vi "Check Python Version.vi"(11 "error in (no error)":errorcluster) -> (4 "standard output":string, 6 "Valid Version?":bool, 15 "error out":errorcluster)   [LabVIEW 2021, in "Measurement Builder.lvlib"]
uses:
  Measurement Builder.lvlib
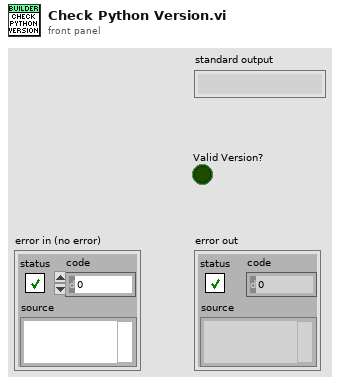
[diagram p1: front panel]
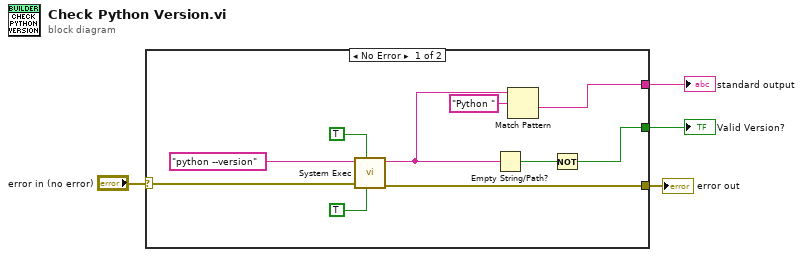
[diagram p0: block diagram]
diagram:
  n1 = case shown="No Error" "error in (no error)" {
    selector: "error in (no error)" -> [w11 w15]
    tunnel: [w10 w15] -> w4
    tunnel: [w5 _] -> w2
    tunnel: [w7 _] -> w1
    frame No Error {
      n2 = call <vilib>:"System Exec.vi"("run minimized? (F)"=TRUE, "wait until completion? (T)"=TRUE, "error in (no error)"=w11, "command line"="python --version") -> ("error out"=w10:errorcluster, "standard output"=w8:string)  [unwired: 4 in, 2 out]
      n3 = Empty String/Path?(string/path=w8) -> (empty?=w9:bool)
      n4 = Match Pattern(string=w8, regular expression="Python ") -> (after substring=w7:string)  [unwired: 1 in, 3 out]
      n5 = Not(x=w9) -> (.not. x?=w5:bool)
    }
    frame Error {
    }
  }
  "error out" <- w4
  "Valid Version?" <- w2
  "standard output" <- w1
